vi "Debug Limit Update.vi"(10 "Slider Values":T1[](array[typedef])) -> ()   [LabVIEW 2013]
uses:
  Logging/Debug Type.ctl
  Limits Widget/Upper Lower Limit Values.ctl
panel:
  # "Lower"
  # "Higher"
  # "Current"
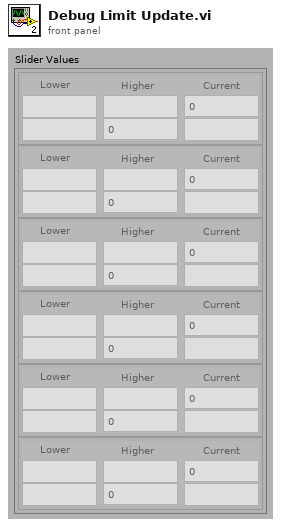
[diagram p1: front panel]
types:
  T1 = typedef "Upper Lower Limit Values.ctl" = cluster{"Global Lo ":dbl, "Local Lo":dbl, "Global Hi ":dbl, "Local Hi ":dbl, "Global Actual":dbl, "Local Actual ":dbl}
  T2 = typedef "Debug Type.ctl" = enum16{"Limit Update", "Limit Change", ""}
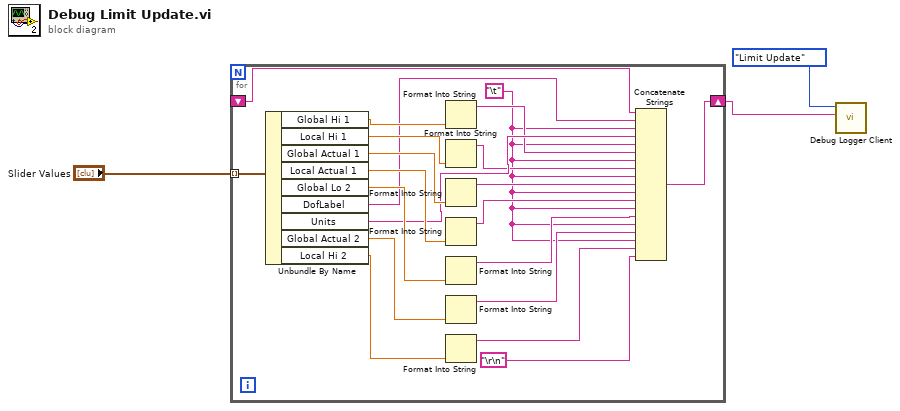
[diagram p0: block diagram]
diagram:
  n1 = for {
    tunnel: "Slider Values" -> [w24] mode=indexing
    shift-right: [w5] -> w2
    shift-left: _ -> [w4]
    w8 = "\t"
    n2 = Unbundle By Name(w24) -> ("Global Hi 1"=w23:dbl, "Local Hi 1"=w22:dbl, "Global Actual 1"=w21:dbl, "Local Actual 1"=w20:dbl, "Global Lo 2"=w19:dbl, "DofLabel"=w16:string, "Units"=w15:string, "Global Actual 2"=w18:dbl, "Local Hi 2"=w17:dbl)
    n3 = Format Into String(w23) -> (resulting string=w14:string)  [unwired: 3 in, 1 out]
    n4 = Format Into String(w22) -> (resulting string=w13:string)  [unwired: 3 in, 1 out]
    n5 = Format Into String(w21) -> (resulting string=w12:string)  [unwired: 3 in, 1 out]
    n6 = Format Into String(w20) -> (resulting string=w11:string)  [unwired: 3 in, 1 out]
    n7 = Format Into String(w19) -> (resulting string=w10:string)  [unwired: 3 in, 1 out]
    n8 = Format Into String(w18) -> (resulting string=w9:string)  [unwired: 3 in, 1 out]
    n9 = Format Into String(w17) -> (resulting string=w7:string)  [unwired: 3 in, 1 out]
    n10 = Concatenate Strings(w4, w16, w8, w15, w8, w14, w8, w13, w8, w12, w8, w11, w8, w10, w8, w9, w8, w7, "\r\n") -> (w5:string)
  }
  n11 = call "Debug Logger Client.vi"("Message"=w2, "Debug Type"=Debug_Type."Limit Update") -> ()  [unwired: 9 in, 1 out]
